vi "rsidr_core_global.vi"() -> ()   [LabVIEW 2015, in "Rohde&Schwarz CMXP NR FR2 Measurement.lvlib"] (continued)
Name"="Fetch Multi Eval Measurement SEM Detected Allocation Results", "Data Type"=enum."RawString", "Command"="FETC:NRMM:MEAS{instance}:MEV:SEM:DALL?", "Access"=enum."Read Only", "Range Table"="", "Read Callback"="", "Write Callback"="", "Range Callback"="", "Check Callback"="", "Rngtable Callback"="", "Coerce Callback"="", "Supported Models"="", "Instrument Options"="", "Check Status Callback"="", "Flags"=0, "Help"="Returns the detected allocation for the measured slot.\n\nAvailable Repeated Capabilities:\ninstance: i0, i1, i2, i3, i4, i5, i6, i7, i8, i9, i10, i11, i12, i13, i14, i15, i16, i17, i18, i19, i20, i21, i22, i23, i24, i25, i26, i27, i28, i29, i30, i31, i32\r\n\nRemote-control command(s):\nFETCh:NRMMw:MEAS<i>:MEValuation:SEMask:DALLocation?"}, {"Level"=4, "Class Only"=FALSE, "Identifier"="RSCMXPNRFR2M_ATTR_FETCH_MULTI_EVAL_MEASUREMENT_ACLR_DETECTED_ALLOCATION", "Descriptive Name"="Fetch Multi Eval Measurement ACLR Detected Allocation", "Data Type"=enum."RawString", "Command"="FETC:NRMM:MEAS{instance}:MEV:ACLR:DALL?", "Access"=enum."Read Only", "Range Table"="", "Read Callback"="", "Write Callback"="", "Range Callback"="", "Check Callback"="", "Rngtable Callback"="", "Coerce Callback"="", "Supported Models"="", "Instrument Options"="", "Check Status Callback"="", "Flags"=0, "Help"="Returns the detected allocation for the measured slot.\n\nAvailable Repeated Capabilities:\ninstance: i0, i1, i2, i3, i4, i5, i6, i7, i8, i9, i10, i11, i12, i13, i14, i15, i16, i17, i18, i19, i20, i21, i22, i23, i24, i25, i26, i27, i28, i29, i30, i31, i32\r\n\nRemote-control command(s):\nFETCh:NRMMw:MEAS<i>:MEValuation:ACLR:DALLocation?"}, {"Level"=3, "Class Only"=TRUE, "Identifier"="", "Descriptive Name"="EVM Trace Results", "Data Type"=enum."ViInt32", "Command"="", "Access"=enum."Read Only", "Range Table"="", "Read Callback"="", "Write Callback"="", "Range Callback"="", "Check Callback"="", "Rngtable Callback"="", "Coerce Callback"="", "Supported Models"="", "Instrument Options"="", "Check Status Callback"="", "Flags"=0, "Help"="Return the EVM trace results of the multi-evaluation measurement"}, {"Level"=4, "Class Only"=FALSE, "Identifier"="RSCMXPNRFR2M_ATTR_READ_MULTI_EVAL_MEASUREMENT_EVM_AVERAGE_RESULTS", "Descriptive Name"="Read Multi Eval Measurement EVM Average Results", "Data Type"=enum."RawString", "Command"="READ:NRMM:MEAS{instance}:MEV:EVM:AVER?", "Access"=enum."Read Only", "Range Table"="", "Read Callback"="", "Write Callback"="", "Range Callback"="", "Check Callback"="", "Rngtable Callback"="", "Coerce Callback"="", "Supported Models"="", "Instrument Options"="", "Check Status Callback"="", "Flags"=0, "Help"="Starts a new single shot measurement and returns the values of the EVM RMS bar graphs for the OFDM symbols in the measured slot.\n\nAvailable Repeated Capabilities:\ninstance: i0, i1, i2, i3, i4, i5, i6, i7, i8, i9, i10, i11, i12, i13, i14, i15, i16, i17, i18, i19, i20, i21, i22, i23, i24, i25, i26, i27, i28, i29, i30, i31, i32\r\n\nRemote-control command(s):\nREAD:NRMMw:MEAS<i>:MEValuation:EVMagnitude:AVERage?"}, {"Level"=4, "Class Only"=FALSE, "Identifier"="RSCMXPNRFR2M_ATTR_READ_MULTI_EVAL_MEASUREMENT_EVM_CURRENT_RESULTS", "Descriptive Name"="Read Multi Eval Measurement EVM Current Results", "Data Type"=enum."RawString", "Command"="READ:NRMM:MEAS{instance}:MEV:EVM:CURR?", "Access"=enum."Read Only", "Range Table"="", "Read Callback"="", "Write Callback"="", "Range Callback"="", "Check Callback"="", "Rngtable Callback"="", "Coerce Callback"="", "Supported Models"="", "Instrument Options"="", "Check Status Callback"="", "Flags"=0, "Help"="Starts a new single shot measurement and returns the values of the EVM RMS bar graphs for the OFDM symbols in the measured slot.\n\nAvailable Repeated Capabilities:\ninstance: i0, i1, i2, i3, i4, i5, i6, i7, i8, i9, i10, i11, i12, i13, i14, i15, i16, i17, i18, i19, i20, i21, i22, i23, i24, i25, i26, i27, i28, i29, i30, i31, i32\r\n\nRemote-control command(s):\nREAD:NRMMw:MEAS<i>:MEValuation:EVMagnitude:CURRent?"}, {"Level"=4, "Class Only"=FALSE, "Identifier"="RSCMXPNRFR2M_ATTR_READ_MULTI_EVAL_MEASUREMENT_EVM_MAXIMUM_RESULTS", "Descriptive Name"="Read Multi Eval Measurement EVM Maximum Results", "Data Type"=enum."RawString", "Command"="READ:NRMM:MEAS{instance}:MEV:EVM:MAX?", "Access"=enum."Read Only", "Range Table"="", "Read Callback"="", "Write Callback"="", "Range Callback"="", "Check Callback"="", "Rngtable Callback"="", "Coerce Callback"="", "Supported Models"="", "Instrument Options"="", "Check Status Callback"="", "Flags"=0, "Help"="Starts a new single shot measurement and returns the values of the EVM RMS bar graphs for the OFDM symbols in the measured slot.\n\nAvailable Repeated Capabilities:\ninstance: i0, i1, i2, i3, i4, i5, i6, i7, i8, i9, i10, i11, i12, i13, i14, i15, i16, i17, i18, i19, i20, i21, i22, i23, i24, i25, i26, i27, i28, i29, i30, i31, i32\r\n\nRemote-control command(s):\nREAD:NRMMw:MEAS<i>:MEValuation:EVMagnitude:MAXimum?"}, {"Level"=4, "Class Only"=FALSE, "Identifier"="RSCMXPNRFR2M_ATTR_FETCH_MULTI_EVAL_MEASUREMENT_EVM_AVERAGE_RESULTS", "Descriptive Name"="Fetch Multi Eval Measurement EVM Average Results", "Data Type"=enum."RawString", "Command"="FETC:NRMM:MEAS{instance}:MEV:EVM:AVER?", "Access"=enum."Read Only", "Range Table"="", "Read Callback"="", "Write Callback"="", "Range Callback"="", "Check Callback"="", "Rngtable Callback"="", "Coerce Callback"="", "Supported Models"="", "Instrument Options"="", "Check Status Callback"="", "Flags"=0, "Help"="Returns the values of the EVM RMS bar graphs for the OFDM symbols in the measured slot.\n\nAvailable Repeated Capabilities:\ninstance: i0, i1, i2, i3, i4, i5, i6, i7, i8, i9, i10, i11, i12, i13, i14, i15, i16, i17, i18, i19, i20, i21, i22, i23, i24, i25, i26, i27, i28, i29, i30, i31, i32\r\n\nRemote-control command(s):\nFETCh:NRMMw:MEAS<i>:MEValuation:EVMagnitude:AVERage?"}, {"Level"=4, "Class Only"=FALSE, "Identifier"="RSCMXPNRFR2M_ATTR_FETCH_MULTI_EVAL_MEASUREMENT_EVM_CURRENT_RESULTS", "Descriptive Name"="Fetch Multi Eval Measurement EVM Current Results", "Data Type"=enum."RawString", "Command"="FETC:NRMM:MEAS{instance}:MEV:EVM:CURR?", "Access"=enum."Read Only", "Range Table"="", "Read Callback"="", "Write Callback"="", "Range Callback"="", "Check Callback"="", "Rngtable Callback"="", "Coerce Callback"="", "Supported Models"="", "Instrument Options"="", "Check Status Callback"="", "Flags"=0, "Help"="Returns the values of the EVM RMS bar graphs for the OFDM symbols in the measured slot.\n\nAvailable Repeated Capabilities:\ninstance: i0, i1, i2, i3, i4, i5, i6, i7, i8, i9, i10, i11, i12, i13, i14, i15, i16, i17, i18, i19, i20, i21, i22, i23, i24, i25, i26, i27, i28, i29, i30, i31, i32\r\n\nRemote-control command(s):\nFETCh:NRMMw:MEAS<i>:MEValuation:EVMagnitude:CURRent?"}, {"Level"=4, "Class Only"=FALSE, "Identifier"="RSCMXPNRFR2M_ATTR_FETCH_MULTI_EVAL_MEASUREMENT_EVM_MAXIMUM_RESULTS", "Descriptive Name"="Fetch Multi Eval Measurement EVM Maximum Results", "Data Type"=enum."RawString", "Command"="FETC:NRMM:MEAS{instance}:MEV:EVM:MAX?", "Access"=enum."Read Only", "Range Table"="", "Read Callback"="", "Write Callback"="", "Range Callback"="", "Check Callback"="", "Rngtable Callback"="", "Coerce Callback"="", "Supported Models"="", "Instrument Options"="", "Check Status Callback"="", "Flags"=0, "Help"="Returns the values of the EVM RMS bar graphs for the OFDM symbols in the measured slot.\n\nAvailable Repeated Capabilities:\ninstance: i0, i1, i2, i3, i4, i5, i6, i7, i8, i9, i10, i11, i12, i13, i14, i15, i16, i17, i18, i19, i20, i21, i22, i23, i24, i25, i26, i27, i28, i29, i30, i31, i32\r\n\nRemote-control command(s):\nFETCh:NRMMw:MEAS<i>:MEValuation:EVMagnitude:MAXimum?"}, {"Level"=4, "Class Only"=FALSE, "Identifier"="RSCMXPNRFR2M_ATTR_READ_MULTI_EVAL_MEASUREMENT_EVM_PEAK_AVERAGE_RESULTS", "Descriptive Name"="Read Multi Eval Measurement EVM Peak Average Results", "Data Type"=enum."RawString", "Command"="READ:NRMM:MEAS{instance}:MEV:EVM:PEAK:AVER?", "Access"=enum."Read Only", "Range Table"="", "Read Callback"="", "Write Callback"="", "Range Callback"="", "Check Callback"="", "Rngtable Callback"="", "Coerce Callback"="", "Supported Models"="", "Instrument Options"="", "Check Status Callback"="", "Flags"=0, "Help"="Starts a new single shot measurement and returns the values of the EVM peak bar graphs for the OFDM symbols in the measured slot.\n\nAvailable Repeated Capabilities:\ninstance: i0, i1, i2, i3, i4, i5, i6, i7, i8, i9, i10, i11, i12, i13, i14, i15, i16, i17, i18, i19, i20, i21, i22, i23, i24, i25, i26, i27, i28, i29, i30, i31, i32\r\n\nRemote-control command(s):\nREAD:NRMMw:MEAS<i>:MEValuation:EVMagnitude:PEAK:AVERage?"}, {"Level"=4, "Class Only"=FALSE, "Identifier"="RSCMXPNRFR2M_ATTR_READ_MULTI_EVAL_MEASUREMENT_EVM_PEAK_CURENT_RESULTS", "Descriptive Name"="Read Multi Eval Measurement EVM Peak Curent Results", "Data Type"=enum."RawString", "Command"="READ:NRMM:MEAS{instance}:MEV:EVM:PEAK:CURR?", "Access"=enum."Read Only", "Range Table"="", "Read Callback"="", "Write Callback"="", "Range Callback"="", "Check Callback"="", "Rngtable Callback"="", "Coerce Callback"="", "Supported Models"="", "Instrument Options"="", "Check Status Callback"="", "Flags"=0, "Help"="Starts a new single shot measurement and returns the values of the EVM peak bar graphs for the OFDM symbols in the measured slot.\n\nAvailable Repeated Capabilities:\ninstance: i0, i1, i2, i3, i4, i5, i6, i7, i8, i9, i10, i11, i12, i13, i14, i15, i16, i17, i18, i19, i20, i21, i22, i23, i24, i25, i26, i27, i28, i29, i30, i31, i32\r\n\nRemote-control command(s):\nREAD:NRMMw:MEAS<i>:MEValuation:EVMagnitude:PEAK:CURRent?"}, {"Level"=4, "Class Only"=FALSE, "Identifier"="RSCMXPNRFR2M_ATTR_READ_MULTI_EVAL_MEASUREMENT_EVM_PEAK_MAXIMUM_RESULTS", "Descriptive Name"="Read Multi Eval Measurement EVM Peak Maximum Results", "Data Type"=enum."RawString", "Command"="READ:NRMM:MEAS{instance}:MEV:EVM:PEAK:MAX?", "Access"=enum."Read Only", "Range Table"="", "Read Callback"="", "Write Callback"="", "Range Callback"="", "Check Callback"="", "Rngtable Callback"="", "Coerce Callback"="", "Supported Models"="", "Instrument Options"="", "Check Status Callback"="", "Flags"=0, "Help"="Starts a new single shot measurement and returns the values of the EVM peak bar graphs for the OFDM symbols in the measured slot.\n\nAvailable Repeated Capabilities:\ninstance: i0, i1, i2, i3, i4, i5, i6, i7, i8, i9, i10, i11, i12, i13, i14, i15, i16, i17, i18, i19, i20, i21, i22, i23, i24, i25, i26, i27, i28, i29, i30, i31, i32\r\n\nRemote-control command(s):\nREAD:NRMMw:MEAS<i>:MEValuation:EVMagnitude:PEAK:MAXimum?"}, {"Level"=4, "Class Only"=FALSE, "Identifier"="RSCMXPNRFR2M_ATTR_FETCH_MULTI_EVAL_MEASUREMENT_EVM_PEAK_AVERAGE_RESULTS", "Descriptive Name"="Fetch Multi Eval Measurement EVM Peak Average Results", "Data Type"=enum."RawString", "Command"="FETC:NRMM:MEAS{instance}:MEV:EVM:PEAK:AVER?", "Access"=enum."Read Only", "Range Table"="", "Read Callback"="", "Write Callback"="", "Range Callback"="", "Check Callback"="", "Rngtable Callback"="", "Coerce Callback"="", "Supported Models"="", "Instrument Options"="", "Check Status Callback"="", "Flags"=0, "Help"="Returns the values of the EVM peak bar graphs for the OFDM symbols in the measured slot.\n\nAvailable Repeated Capabilities:\ninstance: i0, i1, i2, i3, i4, i5, i6, i7, i8, i9, i10, i11, i12, i13, i14, i15, i16, i17, i18, i19, i20, i21, i22, i23, i24, i25, i26, i27, i28, i29, i30, i31, i32\r\n\nRemote-control command(s):\nFETCh:NRMMw:MEAS<i>:MEValuation:EVMagnitude:PEAK:AVERage?"}, {"Level"=4, "Class Only"=FALSE, "Identifier"="RSCMXPNRFR2M_ATTR_FETCH_MULTI_EVAL_MEASUREMENT_EVM_PEAK_CURENT_RESULTS", "Descriptive Name"="Fetch Multi Eval Measurement EVM Peak Curent Results", "Data Type"=enum."RawString", "Command"="FETC:NRMM:MEAS{instance}:MEV:EVM:PEAK:CURR?", "Access"=enum."Read Only", "Range Table"="", "Read Callback"="", "Write Callback"="", "Range Callback"="", "Check Callback"="", "Rngtable Callback"="", "Coerce Callback"="", "Supported Models"="", "Instrument Options"="", "Check Status Callback"="", "Flags"=0, "Help"="Returns the values of the EVM peak bar graphs for the OFDM symbols in the measured slot.\n\nAvailable Repeated Capabilities:\ninstance: i0, i1, i2, i3, i4, i5, i6, i7, i8, i9, i10, i11, i12, i13, i14, i15, i16, i17, i18, i19, i20, i21, i22, i23, i24, i25, i26, i27, i28, i29, i30, i31, i32\r\n\nRemote-control command(s):\nFETCh:NRMMw:MEAS<i>:MEValuation:EVMagnitude:PEAK:CURRent?"}, {"Level"=4, "Class Only"=FALSE, "Identifier"="RSCMXPNRFR2M_ATTR_FETCH_MULTI_EVAL_MEASUREMENT_EVM_PEAK_MAXIMUM_RESULTS", "Descriptive Name"="Fetch Multi Eval Measurement EVM Peak Maximum Results", "Data Type"=enum."RawString", "Command"="FETC:NRMM:MEAS{instance}:MEV:EVM:PEAK:MAX?", "Access"=enum."Read Only", "Range Table"="", "Read Callback"="", "Write Callback"="", "Range Callback"="", "Check Callback"="", "Rngtable Callback"="", "Coerce Callback"="", "Supported Models"="", "Instrument Options"="", "Check Status Callback"="", "Flags"=0, "Help"="Returns the values of the EVM peak bar graphs for the OFDM symbols in the measured slot.\n\nAvailable Repeated Capabilities:\ninstance: i0, i1, i2, i3, i4, i5, i6, i7, i8, i9, i10, i11, i12, i13, i14, i15, i16, i17, i18, i19, i20, i21, i22, i23, i24, i25, i26, i27, i28, i29, i30, i31, i32\r\n\nRemote-control command(s):\nFETCh:NRMMw:MEAS<i>:MEValuation:EVMagnitude:PEAK:MAXimum?"}, {"Level"=4, "Class Only"=FALSE, "Identifier"="RSCMXPNRFR2M_ATTR_READ_MULTI_EVAL_MEASUREMENT_TRACE_EVM_VS_SYMBOL_AVERAGE_RESULTS", "Descriptive Name"="Read Multi Eval Measurement Trace EVM vs Symbol Average Results", "Data Type"=enum."RawString", "Command"="READ:NRMM:MEAS{instance}:MEV:TRAC:EVMS:AVER?", "Access"=enum."Read Only", "Range Table"="", "Read Callback"="", "Write Callback"="", "Range Callback"="", "Check Callback"="", "Rngtable Callback"="", "Coerce Callback"="", "Supported Models"="", "Instrument Options"="", "Check Status Callback"="", "Flags"=0, "Help"="Starts a new single shot measurement and returns the values of the EVM vs modulation symbol trace.\n\nAvailable Repeated Capabilities:\ninstance: i0, i1, i2, i3, i4, i5, i6, i7, i8, i9, i10, i11, i12, i13, i14, i15, i16, i17, i18, i19, i20, i21, i22, i23, i24, i25, i26, i27, i28, i29, i30, i31, i32\r\n\nRemote-control command(s):\nREAD:NRMMw:MEAS<i>:MEValuation:TRACe:EVMSymbol:AVERage?"}, {"Level"=4, "Class Only"=FALSE, "Identifier"="RSCMXPNRFR2M_ATTR_READ_MULTI_EVAL_MEASUREMENT_TRACE_EVM_VS_SYMBOL_CURRENT_RESULTS", "Descriptive Name"="Read Multi Eval Measurement Trace EVM vs Symbol Current Results", "Data Type"=enum."RawString", "Command"="READ:NRMM:MEAS{instance}:MEV:TRAC:EVMS:CURR?", "Access"=enum."Read Only", "Range Table"="", "Read Callback"="", "Write Callback"="", "Range Callback"="", "Check Callback"="", "Rngtable Callback"="", "Coerce Callback"="", "Supported Models"="", "Instrument Options"="", "Check Status Callback"="", "Flags"=0, "Help"="Starts a new single shot measurement and returns the values of the EVM vs modulation symbol trace.\n\nAvailable Repeated Capabilities:\ninstance: i0, i1, i2, i3, i4, i5, i6, i7, i8, i9, i10, i11, i12, i13, i14, i15, i16, i17, i18, i19, i20, i21, i22, i23, i24, i25, i26, i27, i28, i29, i30, i31, i32\r\n\nRemote-control command(s):\nREAD:NRMMw:MEAS<i>:MEValuation:TRACe:EVMSymbol:CURRent?"}, {"Level"=4, "Class Only"=FALSE, "Identifier"="RSCMXPNRFR2M_ATTR_READ_MULTI_EVAL_MEASUREMENT_TRACE_EVM_VS_SYMBOL_MAXIMUM_RESULTS", "Descriptive Name"="Read Multi Eval Measurement Trace EVM vs Symbol Maximum Results", "Data Type"=enum."RawString", "Command"="READ:NRMM:MEAS{instance}:MEV:TRAC:EVMS:MAX?", "Access"=enum."Read Only", "Range Table"="", "Read Callback"="", "Write Callback"="", "Range Callback"="", "Check Callback"="", "Rngtable Callback"="", "Coerce Callback"="", "Supported Models"="", "Instrument Options"="", "Check Status Callback"="", "Flags"=0, "Help"="Starts a new single shot measurement and returns the values of the EVM vs modulation symbol trace.\n\nAvailable Repeated Capabilities:\ninstance: i0, i1, i2, i3, i4, i5, i6, i7, i8, i9, i10, i11, i12, i13, i14, i15, i16, i17, i18, i19, i20, i21, i22, i23, i24, i25, i26, i27, i28, i29, i30, i31, i32\r\n\nRemote-control command(s):\nREAD:NRMMw:MEAS<i>:MEValuation:TRACe:EVMSymbol:MAXimum?"}, {"Level"=4, "Class Only"=FALSE, "Identifier"="RSCMXPNRFR2M_ATTR_FETCH_MULTI_EVAL_MEASUREMENT_TRACE_EVM_VS_SYMBOL_AVERAGE_RESULTS", "Descriptive Name"="Fetch Multi Eval Measurement Trace EVM vs Symbol Average Results", "Data Type"=enum."RawString", "Command"="FETC:NRMM:MEAS{instance}:MEV:TRAC:EVMS:AVER?", "Access"=enum."Read Only", "Range Table"="", "Read Callback"="", "Write Callback"="", "Range Callback"="", "Check Callback"="", "Rngtable Callback"="", "Coerce Callback"="", "Supported Models"="", "Instrument Options"="", "Check Status Callback"="", "Flags"=0, "Help"="Returns the values of the EVM vs modulation symbol trace.\n\nAvailable Repeated Capabilities:\ninstance: i0, i1, i2, i3, i4, i5, i6, i7, i8, i9, i10, i11, i12, i13, i14, i15, i16, i17, i18, i19, i20, i21, i22, i23, i24, i25, i26, i27, i28, i29, i30, i31, i32\r\n\nRemote-control command(s):\nFETCh:NRMMw:MEAS<i>:MEValuation:TRACe:EVMSymbol:AVERage?"}, {"Level"=4, "Class Only"=FALSE, "Identifier"="RSCMXPNRFR2M_ATTR_FETCH_MULTI_EVAL_MEASUREMENT_TRACE_EVM_VS_SYMBOL_CURRENT_RESULTS", "Descriptive Name"="Fetch Multi Eval Measurement Trace EVM vs Symbol Current Results", "Data Type"=enum."RawString", "Command"="FETC:NRMM:MEAS{instance}:MEV:TRAC:EVMS:CURR?", "Access"=enum."Read Only", "Range Table"="", "Read Callback"="", "Write Callback"="", "Range Callback"="", "Check Callback"="", "Rngtable Callback"="", "Coerce Callback"="", "Supported Models"="", "Instrument Options"="", "Check Status Callback"="", "Flags"=0, "Help"="Returns the values of the EVM vs modulation symbol trace.\n\nAvailable Repeated Capabilities:\ninstance: i0, i1, i2, i3, i4, i5, i6, i7, i8, i9, i10, i11, i12, i13, i14, i15, i16, i17, i18, i19, i20, i21, i22, i23, i24, i25, i26, i27, i28, i29, i30, i31, i32\r\n\nRemote-control command(s):\nFETCh:NRMMw:MEAS<i>:MEValuation:TRACe:EVMSymbol:CURRent?"}, {"Level"=4, "Class Only"=FALSE, "Identifier"="RSCMXPNRFR2M_ATTR_FETCH_MULTI_EVAL_MEASUREMENT_TRACE_EVM_VS_SYMBOL_MAXIMUM_RESULTS", "Descriptive Name"="Fetch Multi Eval Measurement Trace EVM vs Symbol Maximum Results", "Data Type"=enum."RawString", "Command"="FETC:NRMM:MEAS{instance}:MEV:TRAC:EVMS:MAX?", "Access"=enum."Read Only", "Range Table"="", "Read Callback"="", "Write Callback"="", "Range Callback"="", "Check Callback"="", "Rngtable Callback"="", "Coerce Callback"="", "Supported Models"="", "Instrument Options"="", "Check Status Callback"="", "Flags"=0, "Help"="Returns the values of the EVM vs modulation symbol trace.\n\nAvailable Repeated Capabilities:\ninstance: i0, i1, i2, i3, i4, i5, i6, i7, i8, i9, i10, i11, i12, i13, i14, i15, i16, i17, i18, i19, i20, i21, i22, i23, i24, i25, i26, i27, i28, i29, i30, i31, i32\r\n\nRemote-control command(s):\nFETCh:NRMMw:MEAS<i>:MEValuation:TRACe:EVMSymbol:MAXimum?"}, {"Level"=4, "Class Only"=FALSE, "Identifier"="RSCMXPNRFR2M_ATTR_READ_MULTI_EVAL_MEASUREMENT_TRACE_EVM_VS_SUBCARRIER_RESULTS", "Descriptive Name"="Read Multi Eval Measurement Trace EVM vs Subcarrier Results", "Data Type"=enum."RawString", "Command"="READ:NRMM:MEAS{instance}:MEV:TRAC:EVMC?", "Access"=enum."Read Only", "Range Table"="", "Read Callback"="", "Write Callback"="", "Range Callback"="", "Check Callback"="", "Rngtable Callback"="", "Coerce Callback"="", "Supported Models"="", "Instrument Options"="", "Check Status Callback"="", "Flags"=0, "Help"="Starts a new single shot measurement and returns the values of the EVM vs subcarrier trace.\n\nAvailable Repeated Capabilities:\ninstance: i0, i1, i2, i3, i4, i5, i6, i7, i8, i9, i10, i11, i12, i13, i14, i15, i16, i17, i18, i19, i20, i21, i22, i23, i24, i25, i26, i27, i28, i29, i30, i31, i32\r\n\nRemote-control command(s):\nREAD:NRMMw:MEAS<i>:MEValuation:TRACe:EVMC?"}, {"Level"=4, "Class Only"=FALSE, "Identifier"="RSCMXPNRFR2M_ATTR_FETCH_MULTI_EVAL_MEASUREMENT_TRACE_EVM_VS_SUBCARRIER_RESULTS", "Descriptive Name"="Fetch Multi Eval Measurement Trace EVM vs Subcarrier Results", "Data Type"=enum."RawString", "Command"="FETC:NRMM:MEAS{instance}:MEV:TRAC:EVMC?", "Access"=enum."Read Only", "Range Table"="", "Read Callback"="", "Write Callback"="", "Range Callback"="", "Check Callback"="", "Rngtable Callback"="", "Coerce Callback"="", "Supported Models"="", "Instrument Options"="", "Check Status Callback"="", "Flags"=0, "Help"="Returns the values of the EVM vs subcarrier trace.\n\nAvailable Repeated Capabilities:\ninstance: i0, i1, i2, i3, i4, i5, i6, i7, i8, i9, i10, i11, i12, i13, i14, i15, i16, i17, i18, i19, i20, i21, i22, i23, i24, i25, i26, i27, i28, i29, i30, i31, i32\r\n\nRemote-control command(s):\nFETCh:NRMMw:MEAS<i>:MEValuation:TRACe:EVMC?"}, {"Level"=3, "Class Only"=TRUE, "Identifier"="", "Descriptive Name"="Magnitude Error", "Data Type"=enum."ViInt32", "Command"="", "Access"=enum."Read Only", "Range Table"="", "Read Callback"="", "Write Callback"="", "Range Callback"="", "Check Callback"="", "Rngtable Callback"="", "Coerce Callback"="", "Supported Models"="", "Instrument Options"="", "Check Status Callback"="", "Flags"=0, "Help"="The following attributes return the values of the magnitude error bar graphs for the OFDM symbols in the measured slot. The results of the current, average and maximum bar graphs can be retrieved."}, {"Level"=4, "Class Only"=FALSE, "Identifier"="RSCMXPNRFR2M_ATTR_READ_MULTI_EVAL_MEASUREMENT_MERR_CURRENT_RESULTS", "Descriptive Name"="Read Multi Eval Measurement Magnitude Error Current Results", "Data Type"=enum."RawString", "Command"="READ:NRMM:MEAS{instance}:MEV:MERR:CURR?", "Access"=enum."Read Only", "Range Table"="", "Read Callback"="", "Write Callback"="", "Range Callback"="", "Check Callback"="", "Rngtable Callback"="", "Coerce Callback"="", "Supported Models"="", "Instrument Options"="", "Check Status Callback"="", "Flags"=0, "Help"="Starts a new single shot measurement and returns the values of the magnitude error bar graphs for the OFDM symbols in the measured slot. The results of the current bar graphs can be retrieved.\n\nAvailable Repeated Capabilities:\ninstance: i0, i1, i2, i3, i4, i5, i6, i7, i8, i9, i10, i11, i12, i13, i14, i15, i16, i17, i18, i19, i20, i21, i22, i23, i24, i25, i26, i27, i28, i29, i30, i31, i32\r\n\nRemote-control command(s):\nREAD:NRMMw:MEAS<i>:MEValuation:MERRor:CURRent?"}, {"Level"=4, "Class Only"=FALSE, "Identifier"="RSCMXPNRFR2M_ATTR_READ_MULTI_EVAL_MEASUREMENT_MERR_AVERAGE_RESULTS", "Descriptive Name"="Read Multi Eval Measurement Magnitude Error Average Results", "Data Type"=enum."RawString", "Command"="READ:NRMM:MEAS{instance}:MEV:MERR:AVER?", "Access"=enum."Read Only", "Range Table"="", "Read Callback"="", "Write Callback"="", "Range Callback"="", "Check Callback"="", "Rngtable Callback"="", "Coerce Callback"="", "Supported Models"="", "Instrument Options"="", "Check Status Callback"="", "Flags"=0, "Help"="Starts a new single shot measurement and returns the values of the magnitude error bar graphs for the OFDM symbols in the measured slot. The results of the average bar graphs can be retrieved.\n\nAvailable Repeated Capabilities:\ninstance: i0, i1, i2, i3, i4, i5, i6, i7, i8, i9, i10, i11, i12, i13, i14, i15, i16, i17, i18, i19, i20, i21, i22, i23, i24, i25, i26, i27, i28, i29, i30, i31, i32\r\n\nRemote-control command(s):\nREAD:NRMMw:MEAS<i>:MEValuation:MERRor:AVERage?"}, {"Level"=4, "Class Only"=FALSE, "Identifier"="RSCMXPNRFR2M_ATTR_READ_MULTI_EVAL_MEASUREMENT_MERR_MAXIMUM_RESULTS", "Descriptive Name"="Read Multi Eval Measurement Magnitude Error Maximum Results", "Data Type"=enum."RawString", "Command"="READ:NRMM:MEAS{instance}:MEV:MERR:MAX?", "Access"=enum."Read Only", "Range Table"="", "Read Callback"="", "Write Callback"="", "Range Callback"="", "Check Callback"="", "Rngtable Callback"="", "Coerce Callback"="", "Supported Models"="", "Instrument Options"="", "Check Status Callback"="", "Flags"=0, "Help"="Starts a new single shot measurement and returns the values of the magnitude error bar graphs for the OFDM symbols in the measured slot. The results of the maximum bar graphs can be retrieved.\n\nAvailable Repeated Capabilities:\ninstance: i0, i1, i2, i3, i4, i5, i6, i7, i8, i9, i10, i11, i12, i13, i14, i15, i16, i17, i18, i19, i20, i21, i22, i23, i24, i25, i26, i27, i28, i29, i30, i31, i32\r\n\nRemote-control command(s):\nREAD:NRMMw:MEAS<i>:MEValuation:MERRor:MAXimum?"}, {"Level"=4, "Class Only"=FALSE, "Identifier"="RSCMXPNRFR2M_ATTR_FETCH_MULTI_EVAL_MEASUREMENT_MERR_CURRENT_RESULTS", "Descriptive Name"="Fetch Multi Eval Measurement Magnitude Error Current Results", "Data Type"=enum."RawString", "Command"="FETC:NRMM:MEAS{instance}:MEV:MERR:CURR?", "Access"=enum."Read Only", "Range Table"="", "Read Callback"="", "Write Callback"="", "Range Callback"="", "Check Callback"="", "Rngtable Callback"="", "Coerce Callback"="", "Supported Models"="", "Instrument Options"="", "Check Status Callback"="", "Flags"=0, "Help"="Returns the values of the magnitude error bar graphs for the OFDM symbols in the measured slot. The results of the current bar graphs can be retrieved.\n\nAvailable Repeated Capabilities:\ninstance: i0, i1, i2, i3, i4, i5, i6, i7, i8, i9, i10, i11, i12, i13, i14, i15, i16, i17, i18, i19, i20, i21, i22, i23, i24, i25, i26, i27, i28, i29, i30, i31, i32\r\n\nRemote-control command(s):\nFETCh:NRMMw:MEAS<i>:MEValuation:MERRor:CURRent?"}, {"Level"=4, "Class Only"=FALSE, "Identifier"="RSCMXPNRFR2M_ATTR_FETCH_MULTI_EVAL_MEASUREMENT_MERR_AVERAGE_RESULTS", "Descriptive Name"="Fetch Multi Eval Measurement Magnitude Error Average Results", "Data Type"=enum."RawString", "Command"="FETC:NRMM:MEAS{instance}:MEV:MERR:AVER?", "Access"=enum."Read Only", "Range Table"="", "Read Callback"="", "Write Callback"="", "Range Callback"="", "Check Callback"="", "Rngtable Callback"="", "Coerce Callback"="", "Supported Models"="", "Instrument Options"="", "Check Status Callback"="", "Flags"=0, "Help"="Returns the values of the magnitude error bar graphs for the OFDM symbols in the measured slot. The results of the average bar graphs can be retrieved.\n\nAvailable Repeated Capabilities:\ninstance: i0, i1, i2, i3, i4, i5, i6, i7, i8, i9, i10, i11, i12, i13, i14, i15, i16, i17, i18, i19, i20, i21, i22, i23, i24, i25, i26, i27, i28, i29, i30, i31, i32\r\n\nRemote-control command(s):\nFETCh:NRMMw:MEAS<i>:MEValuation:MERRor:AVERage?"}, {"Level"=4, "Class Only"=FALSE, "Identifier"="RSCMXPNRFR2M_ATTR_FETCH_MULTI_EVAL_MEASUREMENT_MERR_MAXIMUM_RESULTS", "Descriptive Name"="Fetch Multi Eval Measurement Magnitude Error Maximum Results", "Data Type"=enum."RawString", "Command"="FETC:NRMM:MEAS{instance}:MEV:MERR:MAX?", "Access"=enum."Read Only", "Range Table"="", "Read Callback"="", "Write Callback"="", "Range Callback"="", "Check Callback"="", "Rngtable Callback"="", "Coerce Callback"="", "Supported Models"="", "Instrument Options"="", "Check Status Callback"="", "Flags"=0, "Help"="Returns the values of the magnitude error bar graphs for the OFDM symbols in the measured slot. The results of the maximum bar graphs can be retrieved.\n\nAvailable Repeated Capabilities:\ninstance: i0, i1, i2, i3, i4, i5, i6, i7, i8, i9, i10, i11, i12, i13, i14, i15, i16, i17, i18, i19, i20, i21, i22, i23, i24, i25, i26, i27, i28, i29, i30, i31, i32\r\n\nRemote-control command(s):\nFETCh:NRMMw:MEAS<i>:MEValuation:MERRor:MAXimum?"}, {"Level"=3, "Class Only"=TRUE, "Identifier"="", "Descriptive Name"="Phase Error", "Data Type"=enum."ViInt32", "Command"="", "Access"=enum."Read Only", "Range Table"="", "Read Callback"="", "Write Callback"="", "Range Callback"="", "Check Callback"="", "Rngtable Callback"="", "Coerce Callback"="", "Supported Models"="", "Instrument Options"="", "Check Status Callback"="", "Flags"=0, "Help"="The following attributes return the values of the phase error bar graphs for the OFDM symbols in the measured slot. The results of the current, average and maximum bar graphs can be retrieved."}, {"Level"=4, "Class Only"=FALSE, "Identifier"="RSCMXPNRFR2M_ATTR_READ_MULTI_EVAL_MEASUREMENT_PERR_AVERAGE_RESULTS", "Descriptive Name"="Read Multi Eval Measurement Phase Error Average Results", "Data Type"=enum."RawString", "Command"="READ:NRMM:MEAS{instance}:MEV:PERR:AVER?", "Access"=enum."Read Only", "Range Table"="", "Read Callback"="", "Write Callback"="", "Range Callback"="", "Check Callback"="", "Rngtable Callback"="", "Coerce Callback"="", "Supported Models"="", "Instrument Options"="", "Check Status Callback"="", "Flags"=0, "Help"="Starts a new single shot measurement and returns the values of the phase error bar graphs for the OFDM symbols in the measured slot. The results of the average bar graphs can be retrieved.\n\nAvailable Repeated Capabilities:\ninstance: i0, i1, i2, i3, i4, i5, i6, i7, i8, i9, i10, i11, i12, i13, i14, i15, i16, i17, i18, i19, i20, i21, i22, i23, i24, i25, i26, i27, i28, i29, i30, i31, i32\r\n\nRemote-control command(s):\nREAD:NRMMw:MEAS<i>:MEValuation:PERRor:AVERage?"}, {"Level"=4, "Class Only"=FALSE, "Identifier"="RSCMXPNRFR2M_ATTR_READ_MULTI_EVAL_MEASUREMENT_PERR_CURRENT_RESULTS", "Descriptive Name"="Read Multi Eval Measurement Phase Error Current Results", "Data Type"=enum."RawString", "Command"="READ:NRMM:MEAS{instance}:MEV:PERR:CURR?", "Access"=enum."Read Only", "Range Table"="", "Read Callback"="", "Write Callback"="", "Range Callback"="", "Check Callback"="", "Rngtable Callback"="", "Coerce Callback"="", "Supported Models"="", "Instrument Options"="", "Check Status Callback"="", "Flags"=0, "Help"="Starts a new single shot measurement and returns the values of the phase error bar graphs for the OFDM symbols in the measured slot. The results of the current bar graphs can be retrieved.\n\nAvailable Repeated Capabilities:\ninstance: i0, i1, i2, i3, i4, i5, i6, i7, i8, i9, i10, i11, i12, i13, i14, i15, i16, i17, i18, i19, i20, i21, i22, i23, i24, i25, i26, i27, i28, i29, i30, i31, i32\r\n\nRemote-control command(s):\nREAD:NRMMw:MEAS<i>:MEValuation:PERRor:CURRent?"}, {"Level"=4, "Class Only"=FALSE, "Identifier"="RSCMXPNRFR2M_ATTR_READ_MULTI_EVAL_MEASUREMENT_PERR_MAXIMUM_RESULTS", "Descriptive Name"="Read Multi Eval Measurement Phase Error Maximum Results", "Data Type"=enum."RawString", "Command"="READ:NRMM:MEAS{instance}:MEV:PERR:MAX?", "Access"=enum."Read Only", "Range Table"="", "Read Callback"="", "Write Callback"="", "Range Callback"="", "Check Callback"="", "Rngtable Callback"="", "Coerce Callback"="", "Supported Models"="", "Instrument Options"="", "Check Status Callback"="", "Flags"=0, "Help"="Starts a new single shot measurement and returns the values of the phase error bar graphs for the OFDM symbols in the measured slot. The results of the maximum bar graphs can be retrieved.\n\nAvailable Repeated Capabilities:\ninstance: i0, i1, i2, i3, i4, i5, i6, i7, i8, i9, i10, i11, i12, i13, i14, i15, i16, i17, i18, i19, i20, i21, i22, i23, i24, i25, i26, i27, i28, i29, i30, i31, i32\r\n\nRemote-control command(s):\nREAD:NRMMw:MEAS<i>:MEValuation:PERRor:MAXimum?"}, {"Level"=4, "Class Only"=FALSE, "Identifier"="RSCMXPNRFR2M_ATTR_FETCH_MULTI_EVAL_MEASUREMENT_PERR_AVERAGE_RESULTS", "Descriptive Name"="Fetch Multi Eval Measurement Phase Error Average Results", "Data Type"=enum."RawString", "Command"="FETC:NRMM:MEAS{instance}:MEV:PERR:AVER?", "Access"=enum."Read Only", "Range Table"="", "Read Callback"="", "Write Callback"="", "Range Callback"="", "Check Callback"="", "Rngtable Callback"="", "Coerce Callback"="", "Supported Models"="", "Instrument Options"="", "Check Status Callback"="", "Flags"=0, "Help"="Returns the values of the phase error bar graphs for the OFDM symbols in the measured slot. The results of the average bar graphs can be retrieved.\n\nAvailable Repeated Capabilities:\ninstance: i0, i1, i2, i3, i4, i5, i6, i7, i8, i9, i10, i11, i12, i13, i14, i15, i16, i17, i18, i19, i20, i21, i22, i23, i24, i25, i26, i27, i28, i29, i30, i31, i32\r\n\nRemote-control command(s):\nFETCh:NRMMw:MEAS<i>:MEValuation:PERRor:AVERage?"}, {"Level"=4, "Class Only"=FALSE, "Identifier"="RSCMXPNRFR2M_ATTR_FETCH_MULTI_EVAL_MEASUREMENT_PERR_CURRENT_RESULTS", "Descriptive Name"="Fetch Multi Eval Measurement Phase Error Current Results", "Data Type"=enum."RawString", "Command"="FETC:NRMM:MEAS{instance}:MEV:PERR:CURR?", "Access"=enum."Read Only", "Range Table"="", "Read Callback"="", "Write Callback"="", "Range Callback"="", "Check Callback"="", "Rngtable Callback"="", "Coerce Callback"="", "Supported Models"="", "Instrument Options"="", "Check Status Callback"="", "Flags"=0, "Help"="Returns the values of the phase error bar graphs for the OFDM symbols in the measured slot. The results of the current bar graphs can be retrieved.\n\nAvailable Repeated Capabilities:\ninstance: i0, i1, i2, i3, i4, i5, i6, i7, i8, i9, i10, i11, i12, i13, i14, i15, i16, i17, i18, i19, i20, i21, i22, i23, i24, i25, i26, i27, i28, i29, i30, i31, i32\r\n\nRemote-control command(s):\nFETCh:NRMMw:MEAS<i>:MEValuation:PERRor:CURRent?"}, {"Level"=4, "Class Only"=FALSE, "Identifier"="RSCMXPNRFR2M_ATTR_FETCH_MULTI_EVAL_MEASUREMENT_PERR_MAXIMUM_RESULTS", "Descriptive Name"="Fetch Multi Eval Measurement Phase Error Maximum Results", "Data Type"=enum."RawString", "Command"="FETC:NRMM:MEAS{instance}:MEV:PERR:MAX?", "Access"=enum."Read Only", "Range Table"="", "Read Callback"="", "Write Callback"="", "Range Callback"="", "Check Callback"="", "Rngtable Callback"="", "Coerce Callback"="", "Supported Models"="", "Instrument Options"="", "Check Status Callback"="", "Flags"=0, "Help"="Returns the values of the phase error bar graphs for the OFDM symbols in the measured slot. The results of the maximum bar graphs can be retrieved.\n\nAvailable Repeated Capabilities:\ninstance: i0, i1, i2, i3, i4, i5, i6, i7, i8, i9, i10, i11, i12, i13, i14, i15, i16, i17, i18, i19, i20, i21, i22, i23, i24, i25, i26, i27, i28, i29, i30, i31, i32\r\n\nRemote-control command(s):\nFETCh:NRMMw:MEAS<i>:MEValuation:PERRor:MAXimum?"}, {"Level"=3, "Class Only"=TRUE, "Identifier"="", "Descriptive Name"="Inband Emission", "Data Type"=enum."ViInt32", "Command"="", "Access"=enum."Read Only", "Range Table"="", "Read Callback"="", "Write Callback"="", "Range Callback"="", "Check Callback"="", "Rngtable Callback"="", "Coerce Callback"="", "Supported Models"="", "Instrument Options"="", "Check Status Callback"="", "Flags"=0, "Help"="The following attributes return the values of the inband emissions trace. The current, average and maximum traces can be retrieved."}, {"Level"=4, "Class Only"=FALSE, "Identifier"="RSCMXPNRFR2M_ATTR_READ_MULTI_EVAL_MEASUREMENT_TRACE_IEM_CURRENT_RESULTS", "Descriptive Name"="Read Multi Eval Measurement Trace IEM Current Results", "Data Type"=enum."RawString", "Command"="READ:NRMM:MEAS{instance}:MEV:TRAC:IEM:CURR?", "Access"=enum."Read Only", "Range Table"="", "Read Callback"="", "Write Callback"="", "Range Callback"="", "Check Callback"="", "Rngtable Callback"="", "Coerce Callback"="", "Supported Models"="", "Instrument Options"="", "Check Status Callback"="", "Flags"=0, "Help"="Starts a new single shot measurement and returns the values of the inband emissions trace. The current traces can be retrieved.\n\nAvailable Repeated Capabilities:\ninstance: i0, i1, i2, i3, i4, i5, i6, i7, i8, i9, i10, i11, i12, i13, i14, i15, i16, i17, i18, i19, i20, i21, i22, i23, i24, i25, i26, i27, i28, i29, i30, i31, i32\r\n\nRemote-control command(s):\nREAD:NRMMw:MEAS<i>:MEValuation:TRACe:IEMissions:CURRent?"}, {"Level"=4, "Class Only"=FALSE, "Identifier"="RSCMXPNRFR2M_ATTR_READ_MULTI_EVAL_MEASUREMENT_TRACE_IEM_AVERAGE_RESULTS", "Descriptive Name"="Read Multi Eval Measurement Trace IEM Average Results", "Data Type"=enum."RawString", "Command"="READ:NRMM:MEAS{instance}:MEV:TRAC:IEM:AVER?", "Access"=enum."Read Only", "Range Table"="", "Read Callback"="", "Write Callback"="", "Range Callback"="", "Check Callback"="", "Rngtable Callback"="", "Coerce Callback"="", "Supported Models"="", "Instrument Options"="", "Check Status Callback"="", "Flags"=0, "Help"="Starts a new single shot measurement and returns the values of the inband emissions trace. The average traces can be retrieved.\n\nAvailable Repeated Capabilities:\ninstance: i0, i1, i2, i3, i4, i5, i6, i7, i8, i9, i10, i11, i12, i13, i14, i15, i16, i17, i18, i19, i20, i21, i22, i23, i24, i25, i26, i27, i28, i29, i30, i31, i32\r\n\nRemote-control command(s):\nREAD:NRMMw:MEAS<i>:MEValuation:TRACe:IEMissions:AVERage?"}, {"Level"=4, "Class Only"=FALSE, "Identifier"="RSCMXPNRFR2M_ATTR_READ_MULTI_EVAL_MEASUREMENT_TRACE_IEM_MAXIMUM_RESULTS", "Descriptive Name"="Read Multi Eval Measurement Trace IEM Maximum Results", "Data Type"=enum."RawString", "Command"="READ:NRMM:MEAS{instance}:MEV:TRAC:IEM:MAX?", "Access"=enum."Read Only", "Range Table"="", "Read Callback"="", "Write Callback"="", "Range Callback"="", "Check Callback"="", "Rngtable Callback"="", "Coerce Callback"="", "Supported Models"="", "Instrument Options"="", "Check Status Callback"="", "Flags"=0, "Help"="Starts a new single shot measurement and returns the values of the inband emissions trace. The maximum traces can be retrieved.\n\nAvailable Repeated Capabilities:\ninstance: i0, i1, i2, i3, i4, i5, i6, i7, i8, i9, i10, i11, i12, i13, i14, i15, i16, i17, i18, i19, i20, i21, i22, i23, i24, i25, i26, i27, i28, i29, i30, i31, i32\r\n\nRemote-control command(s):\nREAD:NRMMw:MEAS<i>:MEValuation:TRACe:IEMissions:MAXimum?"}, {"Level"=4, "Class Only"=FALSE, "Identifier"="RSCMXPNRFR2M_ATTR_FETCH_MULTI_EVAL_MEASUREMENT_TRACE_IEM_AVERAGE_RESULTS", "Descriptive Name"="Fetch Multi Eval Measurement Trace IEM Average Results", "Data Type"=enum."RawString", "Command"="FETC:NRMM:MEAS{instance}:MEV:TRAC:IEM:AVER?", "Access"=enum."Read Only", "Range Table"="", "Read Callback"="", "Write Callback"="", "Range Callback"="", "Check Callback"="", "Rngtable Callback"="", "Coerce Callback"="", "Supported Models"="", "Instrument Options"="", "Check Status Callback"="", "Flags"=0, "Help"="Returns the values of the inband emissions trace. The average traces can be retrieved.\n\nAvailable Repeated Capabilities:\ninstance: i0, i1, i2, i3, i4, i5, i6, i7, i8, i9, i10, i11, i12, i13, i14, i15, i16, i17, i18, i19, i20, i21, i22, i23, i24, i25, i26, i27, i28, i29, i30, i31, i32\r\n\nRemote-control command(s):\nFETCh:NRMMw:MEAS<i>:MEValuation:TRACe:IEMissions:AVERage?"}, {"Level"=4, "Class Only"=FALSE, "Identifier"="RSCMXPNRFR2M_ATTR_FETCH_MULTI_EVAL_MEASUREMENT_TRACE_IEM_CURRENT_RESULTS", "Descriptive Name"="Fetch Multi Eval Measurement Trace IEM Current Results", "Data Type"=enum."RawString", "Command"="FETC:NRMM:MEAS{instance}:MEV:TRAC:IEM:CURR?", "Access"=enum."Read Only", "Range Table"="", "Read Callback"="", "Write Callback"="", "Range Callback"="", "Check Callback"="", "Rngtable Callback"="", "Coerce Callback"="", "Supported Models"="", "Instrument Options"="", "Check Status Callback"="", "Flags"=0, "Help"="Returns the values of the inband emissions trace. The current traces can be retrieved.\n\nAvailable Repeated Capabilities:\ninstance: i0, i1, i2, i3, i4, i5, i6, i7, i8, i9, i10, i11, i12, i13, i14, i15, i16, i17, i18, i19, i20, i21, i22, i23, i24, i25, i26, i27, i28, i29, i30, i31, i32\r\n\nRemote-control command(s):\nFETCh:NRMMw:MEAS<i>:MEValuation:TRACe:IEMissions:CURRent?"}, {"Level"=4, "Class Only"=FALSE, "Identifier"="RSCMXPNRFR2M_ATTR_FETCH_MULTI_EVAL_MEASUREMENT_TRACE_IEM_MAXIMUM_RESULTS", "Descriptive Name"="Fetch Multi Eval Measurement Trace IEM Maximum Results", "Data Type"=enum."RawString", "Command"="FETC:NRMM:MEAS{instance}:MEV:TRAC:IEM:MAX?", "Access"=enum."Read Only", "Range Table"="", "Read Callback"="", "Write Callback"="", "Range Callback"="", "Check Callback"="", "Rngtable Callback"="", "Coerce Callback"="", "Supported Models"="", "Instrument Options"="", 
